vi "Post-Build Action.vi"(5 "Files Generated by Build":path[](array[path]), 6 "Top Level/Always Included VIs":path[](array[path]), 7 "Destination Path":path, 8 "error in (no error)":errorcluster, 9 "Target Name":string, 10 "Build Specification Name":string, 11 "Project Path":path) -> (0 "error out":errorcluster)   [LabVIEW 2015, in "BuildVIs.lvlib"]
uses:
  BuildVIs.lvlib
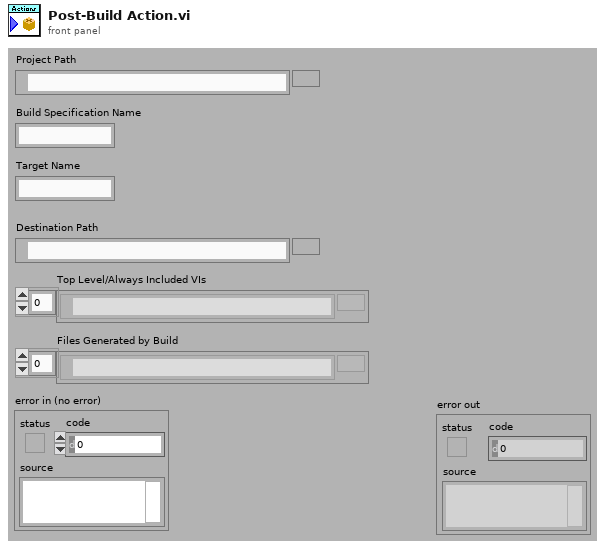
[diagram p1: front panel]
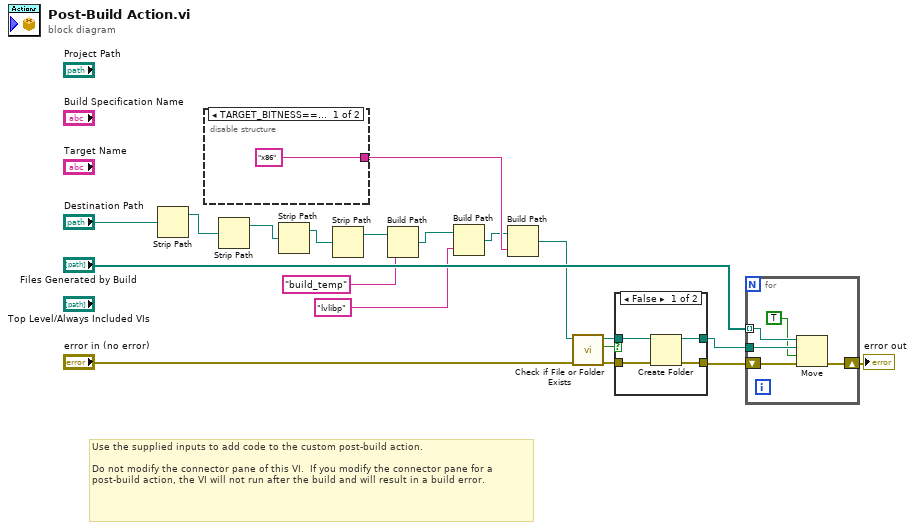
[diagram p0: block diagram]
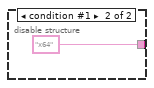
[diagram p3: hidden frame]
diagram:
  # "Use the supplied inputs to add code to the custom post-build action.\n\nDo not modify the connector pane of this VI.  If you modify the connector pane for a post-build action, the VI will not run after the build and will result in a build error."
  n1 = Strip Path(path="Destination Path") -> (stripped path=w10:path)  [unwired: 1 out]
  n2 = disable-structure shown="TARGET_BITNESS==32, Default" {
    disable-tunnel: ["x86" "x64"] -> w5
    frame condition #0 (active) {
    }
    frame condition #1 {
    }
  }
  n3 = Strip Path(path=w10) -> (stripped path=w9:path)  [unwired: 1 out]
  n4 = Strip Path(path=w9) -> (stripped path=w8:path)  [unwired: 1 out]
  n5 = Strip Path(path=w8) -> (stripped path=w7:path)  [unwired: 1 out]
  n6 = Build Path(base path=w7, name or relative path="build_temp") -> (appended path=w4:path)
  n7 = Build Path(base path=w4, name or relative path="lvlibp") -> (appended path=w2:path)
  n8 = Build Path(base path=w2, name or relative path=w5) -> (appended path=w1:path)
  n9 = call <vilib>:"Check if File or Folder Exists.vi"("error in (no error)"="error in (no error)", "path"=w1) -> ("error out"=w18:errorcluster, "file or folder exists?"=w17:bool, "dup path"=w16:path)  [unwired: 7 in]
  n10 = case shown="False" w17 {
    tunnel: w18 -> [w25 w26]
    tunnel: w16 -> [w23 w27]
    tunnel: [w24 w26] -> w15
    tunnel: [w22 w27] -> w13
    frame False {
      n11 = Create Folder(path (use dialog)=w23, error in=w25) -> (created path=w22:path, error out=w24:errorcluster)  [unwired: 1 in, 1 out]
    }
    frame True {
    }
  }
  n12 = for {
    tunnel: w13 -> [w30]
    shift-right: [w31] -> w14
    shift-left: w15 -> [w32]
    tunnel: "Files Generated by Build" -> [w29] mode=indexing
    n13 = Move(source path=w29, error in=w32, 9:TRUE ("overwrite (F)"), 10:w30) -> (error out=w31:errorcluster)  [unwired: 1 in, 2 out]
  }
  "error out" <- w14
